vi "ReadButtonDefinitions.vi"(8 "ErrorIn":errorcluster, 11 "ObjectIn":refnum<class "ButtonCollection.lvclass">) -> (0 "ErrorOut":errorcluster, 2 "ButtonDefinitions":T1[](array[typedef]), 3 "ObjectOut":refnum<class "ButtonCollection.lvclass">)   [LabVIEW 2021, in "ButtonCollection.lvclass"]
uses:
  ButtonCollection.lvclass
  ButtonDefinition.ctl
  ButtonCollection.lvclass/ButtonCollection.ctl
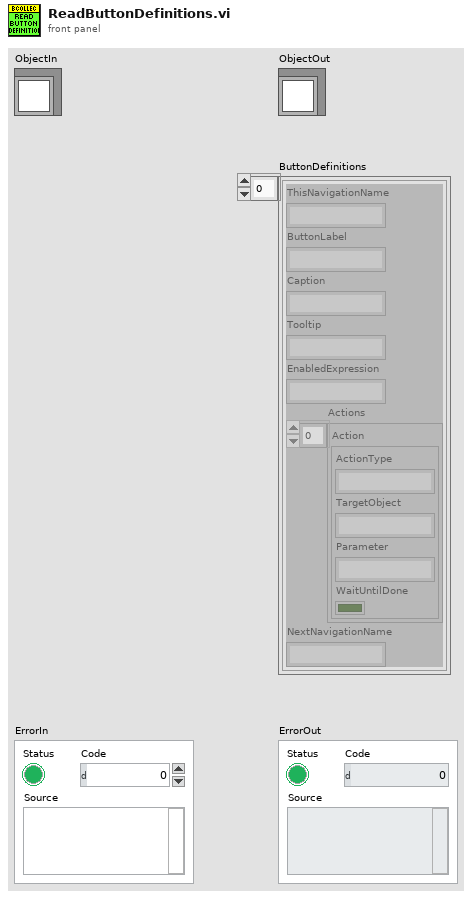
[diagram p1: front panel]
types:
  T1 = typedef "ButtonCollection.lvclass/ButtonDefinition.ctl" = cluster{"ThisNavigationName":string, "ButtonLabel":string, "Caption":string, "Tooltip":string, "EnabledExpression":string, "Actions":cluster{"ActionType":string, "TargetObject":string, "Parameter":string, "WaitUntilDone":bool}[], "NextNavigationName":string}
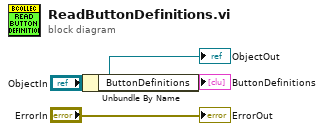
[diagram p0: block diagram]
diagram:
  n1 = Unbundle By Name("ObjectIn") -> ("ButtonDefinitions"=→"ButtonDefinitions":T1[])
  "ErrorOut" <- "ErrorIn"
  "ObjectOut" <- "ObjectIn"
